vi "Dynamic To Waveform Array.vi"(4 "Input":dynamicdata(waveform)) -> (1 "Output":waveform(dbl)[](array[waveform]))   [LabVIEW 2020]
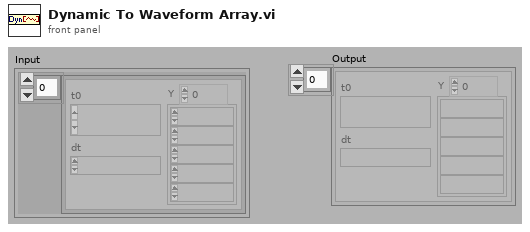
[diagram p1: front panel]
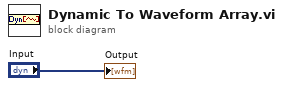
[diagram p0: block diagram]
diagram:
  "Output" <- "Input"
